vi "SetFrontPanelObjectControlValue.vi"(8 "error in (no error)":errorcluster, 9 "Control Name (\"\": Search by Type)":string, 10 "JKI SMO in":refnum<class "JKI SMO.lvclass">, 11 "VI Ref In":refnum<vi>) -> (0 "error out":errorcluster, 3 "VI Ref Out":refnum<vi>)   [LabVIEW 2013, in "JKI SMO.lvclass"]
doc: "Sets the FP control value of an LVClass control, whose type matches the specific type of object in <B>Object in</B> to the value of <B>Object in</B>.\n\n---------------------------------------------------------------\nJKI State Machine Objects™\nhttp://jki.net/state-machine-objects/\nCopyright (C) 2005-2015, JKI <info@jki.net>\nALL RIGHTS RESERVED"
uses:
  JKI SMO.lvclass
panel:
  # "For instructions on how to use the JKI State Machine Objects, examples and video tutorials, visit:\nhttp://jki.net/state-machine-objects/\n\nJKI State Machine Objects™\nhttp://jki.net/state-machine-objects/\nCopyright (C) 2005-2015, JKI <info@jki.net>\nALL RIGHTS RESERVED"
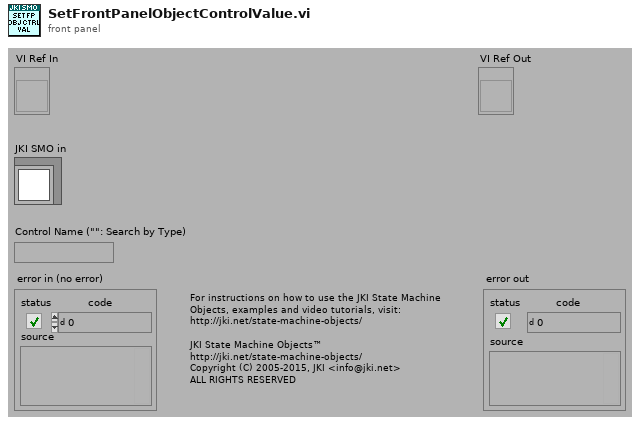
[diagram p1: front panel]
types:
  T1 = enum16{"Set Named Control", "Set Unamed Control", "Exit"}
  T2 = typedef "Type Descriptor Enumeration__ogtk.ctl" = enum8{"<Null>", "I8", "I16", "I32", "I64", "U8", "U16", "U32", "U64", "SGL", "DBL", "EXT", "CSG", "CDB", "CXT", "0x0F", "0x10", "0x11", "0x12", "0x13", "0x14", "Enum U8", "Enum U16", "Enum U32", "Enum U64", "SGL PQ", "DBL PQ", "EXT PQ", "CSG PQ", "CDB PQ", "CXT PQ", "0x1F", "0x20", "Boolean", "0x22", "0x23", "0x24", "0x25", "0x26", "0x27", "0x28", "0x29", "0x2A", "0x2B", "0x2C", "0x2D", "0x2E", "0x2F", "String", "0x31", "Path", "Pict", "0x34", "0x35", "0x36", "DAQ", "0x38", "0x39", "0x3A", "0x3B", "0x3C", "0x3D", "0x3E", "0x3F", "Array", "0x41", "0x42", "0x43", "0x44", "0x45", "0x46", "0x47", "0x48", "0x49", "0x4A", "0x4B", "0x4C", "0x4D", "0x4E", "0x4F", "Cluster", "0x51", "0x52", "Variant", "Waveform", "0x55", "0x56", "0x57", "0x58", "0x59", "0x5A", "0x5B", "0x5C", "0x5D", "0x5E", "0x5F", "0x60", "0x61", "0x62", "0x63", "0x64", "0x65", "0x66", "0x67", "0x68", "0x69", "0x6A", "0x6B", "0x6C", "0x6D", "0x6E", "0x6F", "Refnum"}
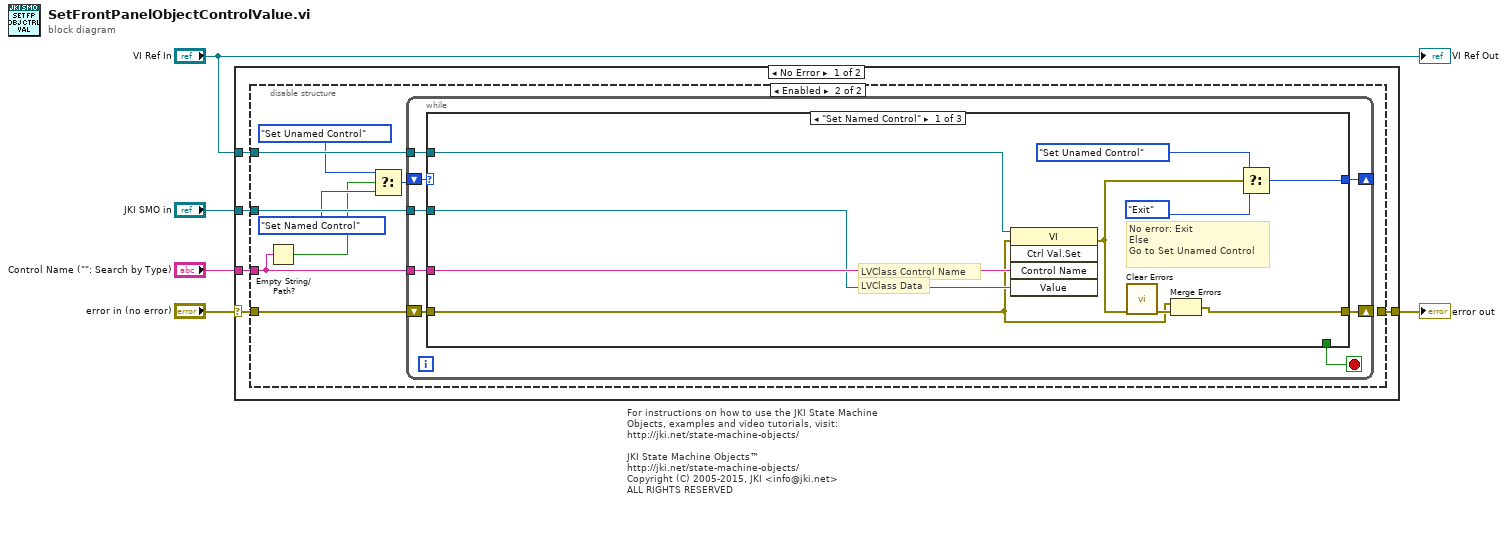
[diagram p0: block diagram]
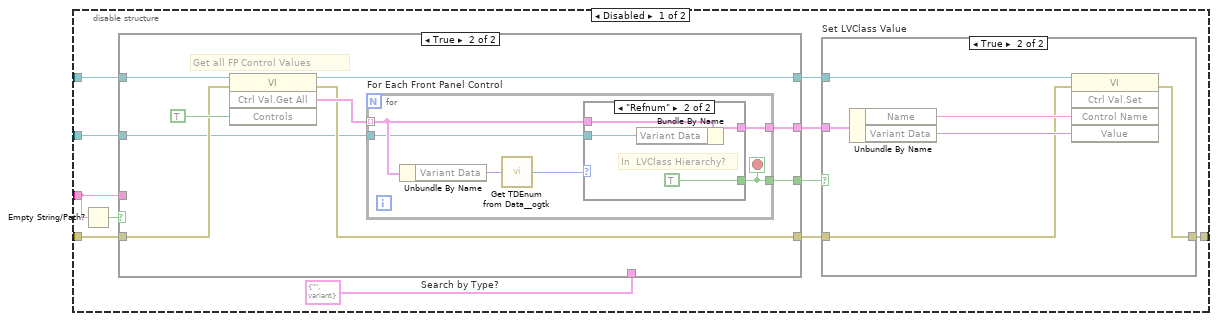
[diagram p2: hidden frame]
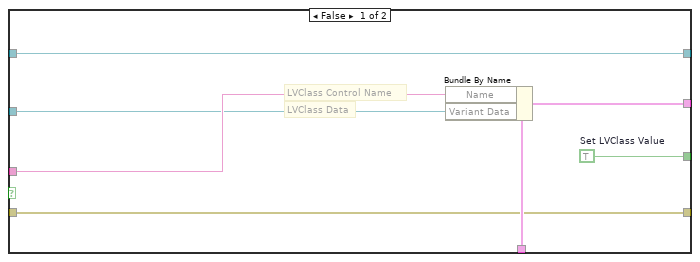
[diagram p3: hidden frame]
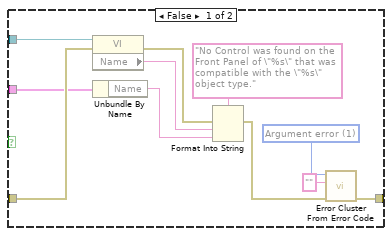
[diagram p5: hidden frame]
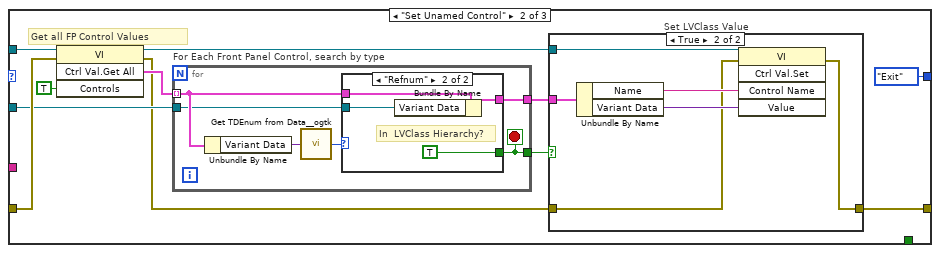
[diagram p6: hidden frame]
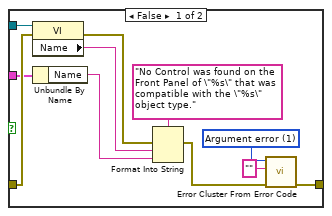
[diagram p7: hidden frame]
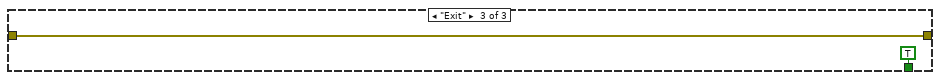
[diagram p9: hidden frame]
diagram:
  # "For instructions on how to use the JKI State Machine Objects, examples and video tutorials, visit:\nhttp://jki.net/state-machine-objects/\n\nJKI State Machine Objects™\nhttp://jki.net/state-machine-objects/\nCopyright (C) 2005-2015, JKI <info@jki.net>\nALL RIGHTS RESERVED"
  n1 = case shown="No Error" "error in (no error)" {
    selector: "error in (no error)" -> [w8 w133]
    tunnel: "JKI SMO in" -> [w6 _]
    tunnel: [w10 w133] -> w3
    tunnel: "VI Ref In" -> [w9 _]
    tunnel: "Control Name (\"\": Search by Type)" -> [w7 _]
    frame No Error {
      n2 = disable-structure shown="Enabled" {
        disable-tunnel: [w21 _] -> w10
        disable-tunnel: w9 -> [w20 w73]
        disable-tunnel: w8 -> [w19 w71]
        disable-tunnel: w7 -> [w18 w66]
        disable-tunnel: w6 -> [w17 w72]
        frame Disabled {
          n3 = Empty String/Path?(string/path=w18) -> (empty?=w12:bool)
          n4 = case "Search by Type?" shown="True" w12 {
            tunnel: [w26 w35] -> w16
            tunnel: [w28 w34] -> w15
            tunnel: [w23 w33] -> w14
            tunnel: w20 -> [w23 w32]
            tunnel: w19 -> [w24 w30]
            tunnel: [w24 w31] -> w13
            tunnel: w18 -> [w27 _]
            tunnel: w17 -> [w22 w29]
            tunnel: cluster{"Name":string, "Variant Data":variant} {"Name"="", "Variant Data"=variant} -> [w25 _]
            frame False {
              w26 = TRUE  # Set LVClass Value
              # "LVClass Control Name"
              # "LVClass Data"
              n5 = Bundle By Name(cluster=w25, "Name"=w27, "Variant Data"=w22) -> (w28:cluster{"Name":string, "Variant Data":variant})
            }
            frame True {
              # "Get all FP Control Values"
              n6 = invoke class="VI" method="Ctrl Val.Get All"(reference=w32, error in=w30, "Controls"=TRUE) -> (reference out=w33:refnum<vi>, error out=w31:errorcluster, "Get All Control Values Variant"=w36:cluster{"Name":string, "Variant Data":variant}[])  [unwired: 1 in, 1 out]
              n7 = for "For Each Front Panel Control" {
                tunnel: w36 -> [w41] mode=indexing
                tunnel: [w40] -> w34
                tunnel: [w42] -> w35
                tunnel: w29 -> [w39]
                stop <- w42 stop-if-true
                n8 = Unbundle By Name(w41) -> ("Variant Data"=w43:variant)
                n9 = call <userlib>:"Get TDEnum from Data__ogtk.vi"("Data"=w43) -> ("Type Descriptor Enumeration"=w38:T2)  [unwired: 4 in]
                n10 = case shown="\"Refnum\"" w38 {
                  tunnel: [_ TRUE] -> w42
                  tunnel: w41 -> [w44 w48]
                  tunnel: [w44 w47] -> w40
                  tunnel: w39 -> [_ w45]
                  frame Default {
                  }
                  frame "Refnum" {
                    # "In  LVClass Hierarchy?"
                    n11 = Bundle By Name(cluster=w48, "Variant Data"=w45) -> (w47:cluster{"Name":string, "Variant Data":variant})
                  }
                }
              }
            }
          }
          n12 = case "Set LVClass Value" shown="True" w16 {
            tunnel: w15 -> [w50 w65]
            tunnel: [w59 w62] -> w21
            tunnel: w14 -> [w56 w61]
            tunnel: w13 -> [w51 w60]
            frame False {
              w58 = 1 items=["No error", "Argument error", "Memory is full", "Out of zone", "End of file", "File already open", "Generic file I/O error", "File not found", "File permission error", "Disk is full", "Duplicate path", "Too many files open", "System feature not enabled", "Resource file not found", "Cannot add resource", "Resource not found", "Image not found", "Image memory error", "Pen does not exist", "Config type invalid", "Config token not found", "Config parse error", "Config memory error", "Bad external code format", "Bad external code offset", "External code not present", "Null window", "Destroy window error", "Null menu", "Print aborted", "Bad print record", "Print driver error", "Windows error during printing", "Memory error during printing", "Print dialog error", "Generic print error", "Invalid device refnum", "Device not found", "Device parameter error", "Device unit error", "Cannot open device", "Device call aborted", "Generic error", "Cancelled by user", "Object ID too low", "Object ID too high", "Object not in heap", "Unknown heap", "Unknown object (invalid DefProc)", "Unknown object (DefProc not in table)", "Message out of range", "Invalid (null) method", "Unknown message", "Manager call not supported", "Bad address", "Network operation in progress", "Network operation timed out", "Connection is busy", "Network attribute not supported", "Network error", "Address in use", "System out of memory", "Connection aborted", "Connection refused", "Not connected", "Already connected", "Connection closed", "Initialization error (interapplication manager)", "Bad occurrence", "Wait on unbound occurrence handler", "Occurrence queue overflow", "Datalog type conflict", "Unused", "Unrecognized type (interapplication manager)", "Memory corrupt", "Failed to make temporary DLL", "Old CIN version", "Drag socket not found", "Failed to load drop-object", "Failed to register OLE object", "Failed to release OLE object", "Format specifier type mismatch", "Unknown format specifier", "Too few format specifiers", "Too many format specifiers", "Scan failed", "Newer CIN version", "Error converting to variant", "Runtime menu error", "Password tampered", "Variant attribute not found", "Incompatible variant data type", "Event data is not available", "Event Store is not present", "Occurrence is not found", "Event Queue is not created", "Event info is not available", "Refnum passed is NULL", "Error retrieving Class GUID", "Error retrieving CoClass GUID", "Error retrieving TypeLib GUID.", "Bad built application magic bytes.", "Specific driver is different from the specific driver associated with the Logical Name.", "There is no session opened to the class driver.", "Max Error", "MAX - Error with config objects", "MAX - Error loading configuration", "MAX - Group not supported"]
              n13 = property class="VI"(reference=w56, error in=w51) -> (error out=w53:errorcluster, "Name"=w55:string)  [unwired: 1 out]
              n14 = Unbundle By Name(w50) -> ("Name"=w49:string)
              n15 = Format Into String(format string="No Control was found on the Front Panel of \"%s\" that was compatible with the \"%s\" object type.", error in=w53, w55, w49) -> (error out=w52:errorcluster)  [unwired: 1 in, 1 out]
              n16 = call <vilib>:"Error Cluster From Error Code.vi"("error in (no error)"=w52, "error message (\"\")"="" ("error message (\"\")"), "error code (0)"=w58) -> ("error out"=w59:errorcluster)  [unwired: 1 in, 5 out]
            }
            frame True {
              n17 = Unbundle By Name(w65) -> ("Name"=w64:string, "Variant Data"=w63:variant)
              n18 = invoke class="VI" method="Ctrl Val.Set"(reference=w61, error in=w60, "Control Name"=w64, "Value"=w63) -> (error out=w62:errorcluster)  [unwired: 1 in, 4 out]
            }
          }
        }
        frame Enabled {
          n19 = Empty String/Path?(string/path=w66) -> (empty?=w67:bool)
          n20 = Select(t=T1."Set Unamed Control", s=w67, f=T1."Set Named Control") -> (s? t:f=w70:T1)
          n21 = while {
            tunnel: w73 -> [w75]
            tunnel: w72 -> [w79]
            shift-right: [w77] -> _
            shift-left: w71 -> [w80]
            shift-right: [w76] -> _
            shift-left: w70 -> [w81]
            tunnel: w66 -> [w78]
            stop <- w74 stop-if-true
            n22 = case shown="\"Set Named Control\"" w81 {
              tunnel: w80 -> [w82 w99 w131]
              tunnel: w79 -> [w90 w98 _]
              tunnel: w78 -> [w91 _ _]
              tunnel: [w83 w95 w131] -> w77
              tunnel: [w87 T1."Exit" _] -> w76
              tunnel: w75 -> [w85 w100 _]
              tunnel: [_ _ TRUE] -> w74
              frame "Set Named Control" {
                # "No error: Exit\nElse\nGo to Set Unamed Control"
                # "LVClass Control Name"
                # "LVClass Data"
                n23 = invoke class="VI" method="Ctrl Val.Set"(reference=w85, error in=w82, "Control Name"=w91, "Value"=w90) -> (error out=w89:errorcluster)  [unwired: 1 in, 4 out]
                n24 = call <vilib>:"Clear Errors.vi"("error in (no error)"=w89) -> ("error out"=w84:errorcluster)  [unwired: 6 in]
                n25 = Merge Errors(w82, w84) -> (w83:errorcluster)
                n26 = Select(t=T1."Set Unamed Control", s=w89, f=T1."Exit") -> (s? t:f=w87:T1)
              }
              frame "Set Unamed Control" {
                # "Get all FP Control Values"
                n27 = invoke class="VI" method="Ctrl Val.Get All"(reference=w100, error in=w99, "Controls"=TRUE) -> (reference out=w93:refnum<vi>, error out=w96:errorcluster, "Get All Control Values Variant"=w101:cluster{"Name":string, "Variant Data":variant}[])  [unwired: 1 in, 1 out]
                n28 = for "For Each Front Panel Control, search by type" {
                  tunnel: w101 -> [w123] mode=indexing
                  tunnel: [w122] -> w94
                  tunnel: [w124] -> w92
                  tunnel: w98 -> [w121]
                  stop <- w124 stop-if-true
                  n29 = Unbundle By Name(w123) -> ("Variant Data"=w125:variant)
                  n30 = call <userlib>:"Get TDEnum from Data__ogtk.vi"("Data"=w125) -> ("Type Descriptor Enumeration"=w120:T2)  [unwired: 4 in]
                  n31 = case shown="\"Refnum\"" w120 {
                    tunnel: [_ TRUE] -> w124
                    tunnel: w123 -> [w126 w130]
                    tunnel: [w126 w129] -> w122
                    tunnel: w121 -> [_ w127]
                    frame Default {
                    }
                    frame "Refnum" {
                      # "In  LVClass Hierarchy?"
                      n32 = Bundle By Name(cluster=w130, "Variant Data"=w127) -> (w129:cluster{"Name":string, "Variant Data":variant})
                    }
                  }
                }
                n33 = case "Set LVClass Value" shown="True" w92 {
                  tunnel: w94 -> [w104 w119]
                  tunnel: [w113 w116] -> w95
                  tunnel: w93 -> [w110 w115]
                  tunnel: w96 -> [w105 w114]
                  frame False {
                    w112 = 1 items=["No error", "Argument error", "Memory is full", "Out of zone", "End of file", "File already open", "Generic file I/O error", "File not found", "File permission error", "Disk is full", "Duplicate path", "Too many files open", "System feature not enabled", "Resource file not found", "Cannot add resource", "Resource not found", "Image not found", "Image memory error", "Pen does not exist", "Config type invalid", "Config token not found", "Config parse error", "Config memory error", "Bad external code format", "Bad external code offset", "External code not present", "Null window", "Destroy window error", "Null menu", "Print aborted", "Bad print record", "Print driver error", "Windows error during printing", "Memory error during printing", "Print dialog error", "Generic print error", "Invalid device refnum", "Device not found", "Device parameter error", "Device unit error", "Cannot open device", "Device call aborted", "Generic error", "Cancelled by user", "Object ID too low", "Object ID too high", "Object not in heap", "Unknown heap", "Unknown object (invalid DefProc)", "Unknown object (DefProc not in table)", "Message out of range", "Invalid (null) method", "Unknown message", "Manager call not supported", "Bad address", "Network operation in progress", "Network operation timed out", "Connection is busy", "Network attribute not supported", "Network error", "Address in use", "System out of memory", "Connection aborted", "Connection refused", "Not connected", "Already connected", "Connection closed", "Initialization error (interapplication manager)", "Bad occurrence", "Wait on unbound occurrence handler", "Occurrence queue overflow", "Datalog type conflict", "Unused", "Unrecognized type (interapplication manager)", "Memory corrupt", "Failed to make temporary DLL", "Old CIN version", "Drag socket not found", "Failed to load drop-object", "Failed to register OLE object", "Failed to release OLE object", "Format specifier type mismatch", "Unknown format specifier", "Too few format specifiers", "Too many format specifiers", "Scan failed", "Newer CIN version", "Error converting to variant", "Runtime menu error", "Password tampered", "Variant attribute not found", "Incompatible variant data type", "Event data is not available", "Event Store is not present", "Occurrence is not found", "Event Queue is not created", "Event info is not available", "Refnum passed is NULL", "Error retrieving Class GUID", "Error retrieving CoClass GUID", "Error retrieving TypeLib GUID.", "Bad built application magic bytes.", "Specific driver is different from the specific driver associated with the Logical Name.", "There is no session opened to the class driver.", "Max Error", "MAX - Error with config objects", "MAX - Error loading configuration", "MAX - Group not supported"]
                    n34 = property class="VI"(reference=w110, error in=w105) -> (error out=w107:errorcluster, "Name"=w109:string)  [unwired: 1 out]
                    n35 = Unbundle By Name(w104) -> ("Name"=w103:string)
                    n36 = Format Into String(format string="No Control was found on the Front Panel of \"%s\" that was compatible with the \"%s\" object type.", error in=w107, w109, w103) -> (error out=w106:errorcluster)  [unwired: 1 in, 1 out]
                    n37 = call <vilib>:"Error Cluster From Error Code.vi"("error in (no error)"=w106, "error message (\"\")"="" ("error message (\"\")"), "error code (0)"=w112) -> ("error out"=w113:errorcluster)  [unwired: 1 in, 5 out]
                  }
                  frame True {
                    n38 = Unbundle By Name(w119) -> ("Name"=w118:string, "Variant Data"=w117:variant)
                    n39 = invoke class="VI" method="Ctrl Val.Set"(reference=w115, error in=w114, "Control Name"=w118, "Value"=w117) -> (error out=w116:errorcluster)  [unwired: 1 in, 4 out]
                  }
                }
              }
              frame "Exit" {
              }
            }
          }
        }
      }
    }
    frame Error {
    }
  }
  "error out" <- w3
  "VI Ref Out" <- "VI Ref In"
